vi "Register Listener.vi"(8 "Error In":errorcluster, 11 "Listener ID":string) -> (0 "Error Out":errorcluster)   [LabVIEW 2017, in "Logger.lvlib"]
doc: "Creates a new listener for logging statements. By default, there is at least one listener, which is the internal listener used for the default log file."
uses:
  Logger.lvlib
  Private/Action.ctl
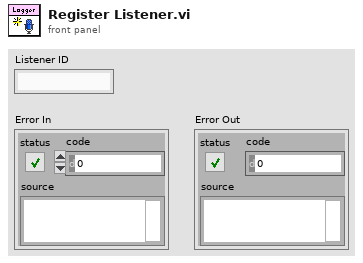
[diagram p1: front panel]
types:
  T1 = typedef "Logger.lvlib/Action.ctl" = enum16{"Initialize", "Register", "Log", "Unregister", "Set Level", "Shutdown"}
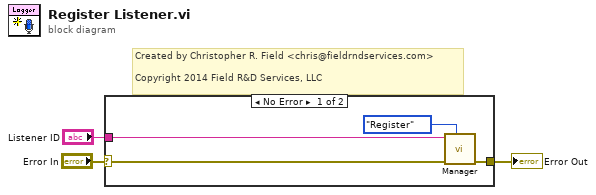
[diagram p0: block diagram]
diagram:
  # "Created by Christopher R. Field <chris@fieldrndservices.com>\n\nCopyright 2014 Field R&D Services, LLC"
  n1 = case shown="No Error" "Error In" {
    selector: "Error In" -> [w6 w8]
    tunnel: "Listener ID" -> [w5 _]
    tunnel: [w4 w8] -> w1
    frame No Error {
      n2 = call "Manager.vi"("Action"=Action."Register", "Error In"=w6, "Value In"=w5) -> ("Error Out"=w4:errorcluster)  [unwired: 8 in]
    }
    frame Error {
    }
  }
  "Error Out" <- w1
